vi "FindFreePosition.vi"(0 "reference":refnum<class "Graph.lvclass">, 1 "NodePointIn":T1 {"y" format="%.2f"; "x" format="%.2f"}, 2 "Node":refnum<class "AbstractNode.lvclass">, 5 "error in (no error)":errorcluster) -> (14 "reference out":refnum<class "Graph.lvclass">, 15 "NodePointOut":T1 {"y" format="%.2f"; "x" format="%.2f"}, 19 "error out":errorcluster)   [LabVIEW 2020, in "Graph.lvclass"]
doc: "Finds a node containing the given point.\n @param p a point\n @return a node containing p or null if no nodes contain p\n */\n public Node findNode(Point2D p)"
uses:
  <resource>/Framework/Providers/Open_GDS/UML/Graph_class/Graph.lvclass
  <resource>/Framework/Providers/Open_GDS/UML/General/Point/Point Point2D.ctl
  <resource>/Framework/Providers/Open_GDS/UML/AbstractNode_class/AbstractNode.lvclass
  <resource>/Framework/Providers/Open_GDS/UML/General/Rectangle/Rectangle DirectionToTest.ctl
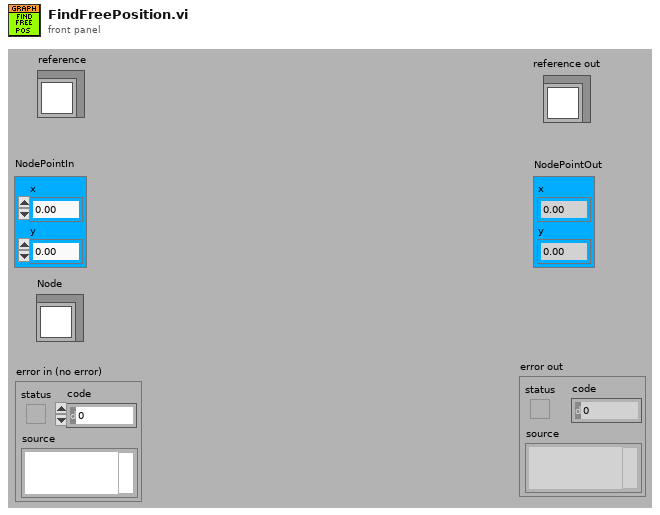
[diagram p1: front panel]
types:
  T1 = typedef "Point Point2D.ctl" = cluster{"x":dbl, "y":dbl}
  T2 = typedef "Rectangle DirectionToTest.ctl" = enum16{"E-S-W-N", "ES-S-WS"}
  T3 = typedef "Rectangle Rectangle2D.ctl" = cluster{"x":dbl, "y":dbl, "width":dbl, "height":dbl}
  T4 = typedef "Graph.lvclass/ObjectAttributes.ctl" = cluster{"nodes":refnum<class "AbstractNode.lvclass">[], "edges":refnum<class "AbstractEdge.lvclass">[], "nodesToBeRemoved":refnum<class "AbstractNode.lvclass">[], "edgesToBeRemoved":refnum<class "AbstractEdge.lvclass">[], "needsLayout":bool, "LayoutNodes":refnum<class "AbstractNode.lvclass">[]}
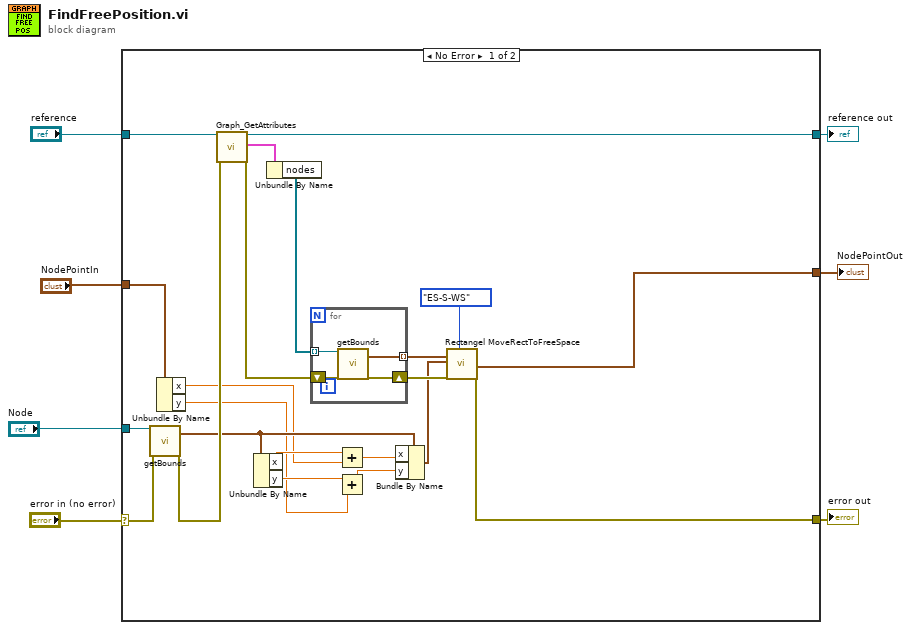
[diagram p0: block diagram]
diagram:
  n1 = case shown="No Error" "error in (no error)" {
    selector: "error in (no error)" -> [w22 w35]
    tunnel: "reference" -> [w29 w36]
    tunnel: [w11 w35] -> w6
    tunnel: [w28 w36] -> w5
    tunnel: "NodePointIn" -> [w20 w34]
    tunnel: "Node" -> [w23 _]
    tunnel: [w10 w34] -> w1
    frame No Error {
      n2 = call-dynamic "getBounds.vi"("reference"=w23, "error in (no error)"=w22) -> ("bounds"=w18:T3, "error out"=w21:errorcluster)  [unwired: 16 out]
      n3 = Unbundle By Name(w20) -> ("x"=w16:dbl, "y"=w14:dbl)
      n4 = call <resource>:"Graph_GetAttributes.vi"("reference in"=w29, "error in (no error)"=w21) -> ("reference out"=w28:refnum<class "Graph.lvclass">, "Data"=w8:T4, "error out"=w26:errorcluster)  [unwired: 1 in, 14 out]
      n5 = Unbundle By Name(w18) -> ("x"=w17:dbl, "y"=w15:dbl)
      n6 = Unbundle By Name(w8) -> ("nodes"=w27:refnum<class "AbstractNode.lvclass">[])
      n7 = for {
        tunnel: w27 -> [w33] mode=indexing
        shift-right: [w31] -> w24
        shift-left: w26 -> [w32]
        tunnel: [w30] -> w25 mode=indexing
        n8 = call-dynamic "getBounds.vi"("reference"=w33, "error in (no error)"=w32) -> ("bounds"=w30:T3, "error out"=w31:errorcluster)  [unwired: 16 out]
      }
      n9 = Add(x=w17, y=w16) -> (x+y=w13:dbl)
      n10 = Add(x=w15, y=w14) -> (x+y=w12:dbl)
      n11 = Bundle By Name(cluster=w18, "x"=w13, "y"=w12) -> (w19:T3)
      n12 = call <resource>:"Rectangel MoveRectToFreeSpace.vi"("BoundsArray"=w25, "bounds"=w19, "error in (no error)"=w24, "DirectionsToTest(E-S-W-N)"=Rectangle_DirectionToTest."ES-S-WS") -> ("point"=w10:T1, "error out"=w11:errorcluster)  [unwired: 14 out]
    }
    frame Error {
    }
  }
  "reference out" <- w5
  "error out" <- w6
  "NodePointOut" <- w1
